vi "Get Selected Experiment.vi"(8 "error in":errorcluster, 11 "Experiments ref":refnum<vi>) -> (0 "error out":errorcluster, 1 "URL":string, 2 "Experiment":T1, 3 "Experiments ref out":refnum<vi>)   [LabVIEW 2020]
uses:
  Utilities/iCalendar/Extract iCalendar String.ctl
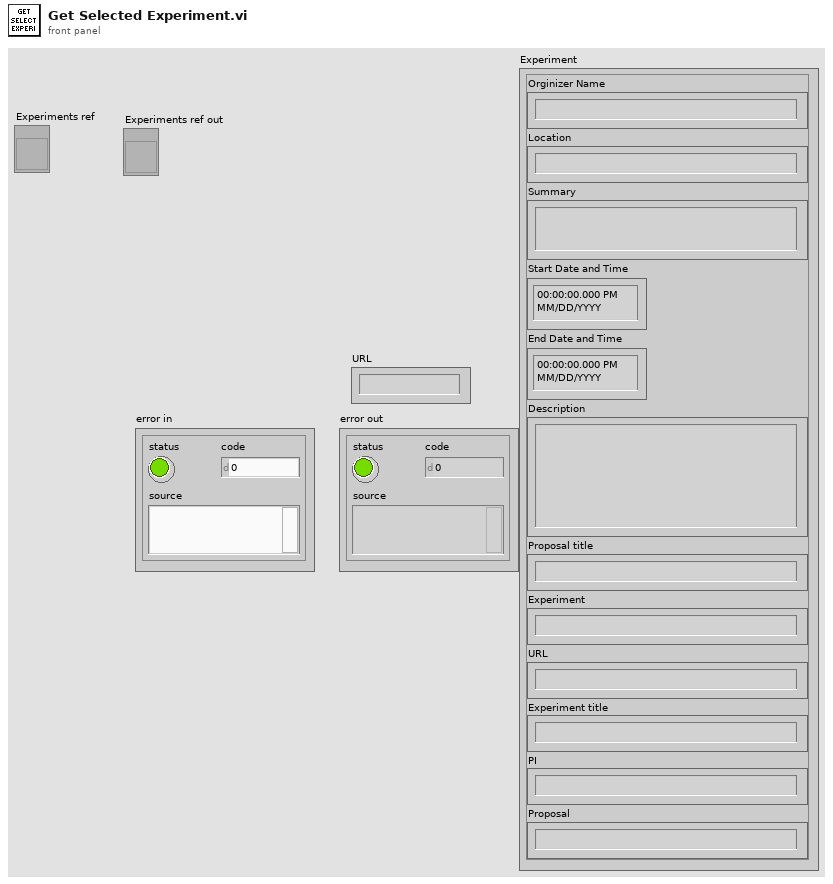
[diagram p1: front panel]
types:
  T1 = typedef "Extract iCalendar String.ctl" = cluster{"Orginizer Name":string, "Location":string, "Summary":string, "Start Date and Time":timestamp, "End Date and Time":timestamp, "Description":string, "Proposal title":string, "Experiment":string, "URL":string, "Experiment title":string, "PI":string, "Proposal":string}
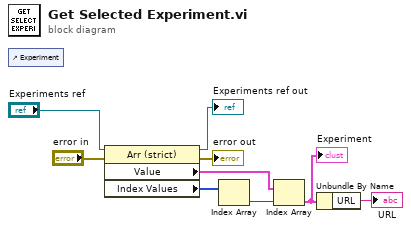
[diagram p0: block diagram]
diagram:
  n1 = control-ref of="Experiment"() -> ()  [unwired: 1 out]
  n2 = property class="Arr (strict)"(reference="Experiments ref", error in="error in") -> (reference out=→"Experiments ref out":refnum<vi>, error out=→"error out":errorcluster, "Value"=w7:T1[], "Index Values"=w8:u32[])
  n3 = Index Array(array=w8) -> (element=w6:u32)  [unwired: 1 in]
  n4 = Index Array(array=w7, index=w6) -> (element=w4:T1)
  "Experiment" <- w4
  n5 = Unbundle By Name(w4) -> ("URL"=→"URL":string)
